vi "csm_lumikki_instron_startLogging_poller.vi"() -> ()   [LabVIEW 2009]
uses:
  <vilib>/Utility/file.llb/Write To Spreadsheet File (DBL).vi
panel:
  in  "Interval/Buffer Parameters":T1={"Sample interval - ms (2)"=2.0, "Buffer Length (1000)"=1000, "No. of Buffers (0)"=0} {"Sample interval - ms (2)" min=0.2 format="%.1f"}
  out "Waveform Graph 2":dbl[][](graph)
  # "datalogger internal \npreferences:"
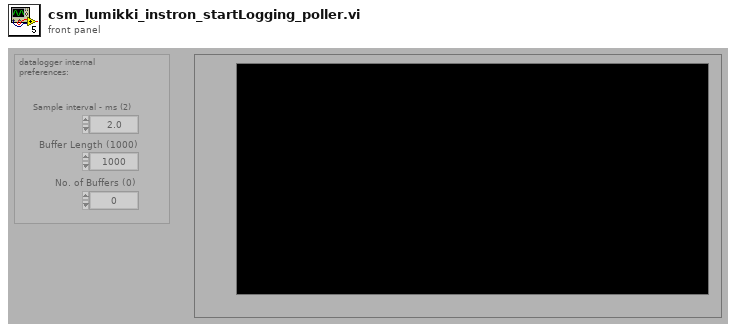
[diagram p1: front panel]
types:
  T1 = cluster{"Sample interval - ms (2)":dbl, "Buffer Length (1000)":i32, "No. of Buffers (0)":i32}
  T2 = cluster{"Device ID":i32, "Device Name":string, "Device Type":i32}[]
  T3 = typedef "NI_Matrix.lvlib/RealMatrix.ctl" = dbl[][]
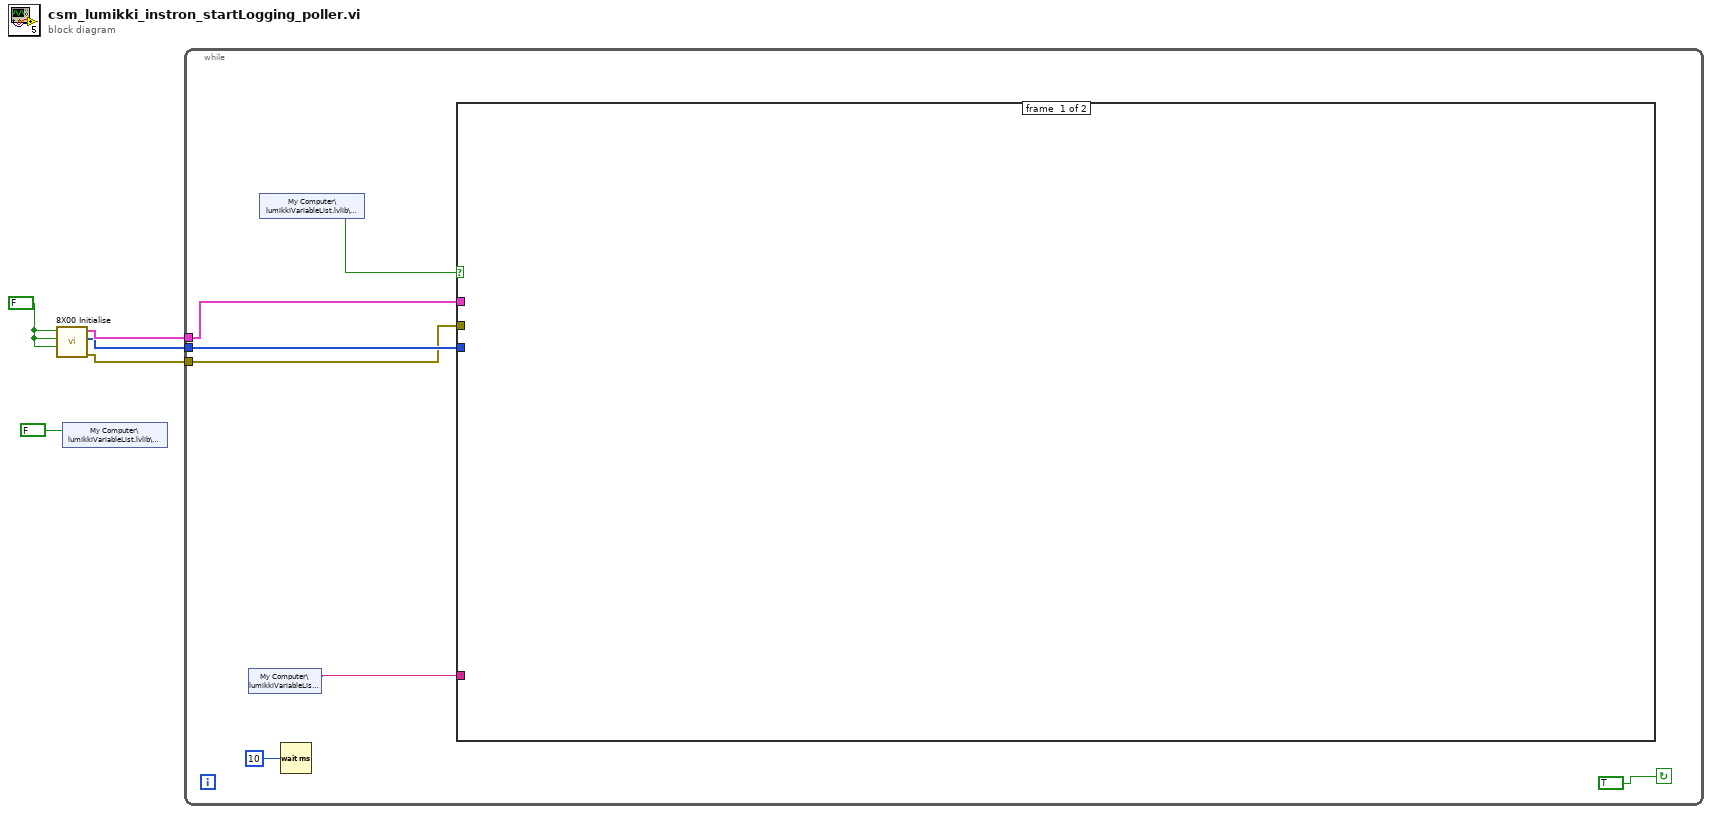
[diagram p0: block diagram]
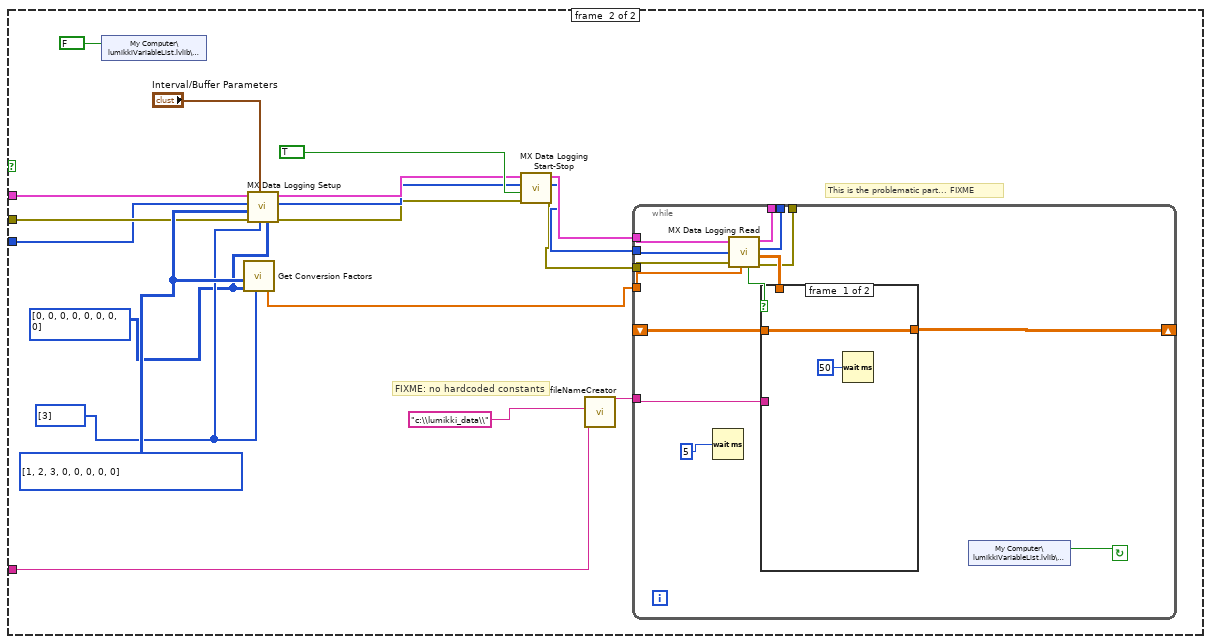
[diagram p2: hidden frame]
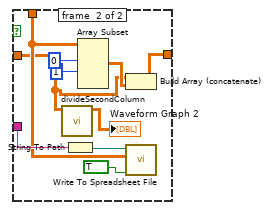
[diagram p3: hidden frame]
diagram:
  w5 = FALSE ("Create Console? (T)")
  n1 = call "8X00 Initialise.vi"("Reset?"=w5, "Create DVM? (T)"=w5, "Create Console? (T)"=w5) -> ("error out"=w2:errorcluster, "Axis Selector"=w3:i32[], "Axis Information"=w4:T2)  [unwired: 1 in, 1 out]
  n2 = shared-variable "My Computer\\lumikkiVariableList.lvlib\\startLogging"(FALSE ("startLogging")) -> ()  [unwired: 1 in, 1 out]
  n3 = while {
    tunnel: w4 -> [w10]
    tunnel: w3 -> [w9]
    tunnel: w2 -> [w8]
    stop <- TRUE continue-if-true
    n4 = shared-variable "My Computer\\lumikkiVariableList.lvlib\\expId"() -> (w6:string)  [unwired: 1 in, 1 out]
    n5 = shared-variable "My Computer\\lumikkiVariableList.lvlib\\startLogging"() -> (w7:bool)  [unwired: 1 in, 1 out]
    n6 = Wait (ms)(milliseconds to wait=u32 10) -> ()  [unwired: 1 out]
    n7 = case shown="True" w7 {
      tunnel: w10 -> [_ w16]
      tunnel: w9 -> [_ w17]
      tunnel: w8 -> [_ w18]
      tunnel: w6 -> [_ w15]
      frame #0 {
      }
      frame #1 {
        w28 = i32[] [3] ("Number of Columns")
        w27 = i32[][] [[0, 0, 0, 0, 0, 0, 0, 0]] items=["Feedback", "Direct Auxilary"] ("Column Types")
        w29 = i32[][] [[1, 2, 3, 0, 0, 0, 0, 0]] items=["Not Used", "Channel 1/Logging time", "Channel 2/Controlling command", "Channel 3/Controlling error", "Channel 4/Elapsed quarter-cycle counter", "Total accumulated quarter-cycle counter", "Elapsed segment counter", "Total accumulated segment counter", "Servovalve drive", "Block count", "Uncompensated servovalve drive", "Geometric compensation output 1", "Geometric compensation output 2", "Re-Sampling Filter 1", "Re-Sampling Filter 2", "Re-Sampling Filter 3", "Re-Sampling Filter 4", "Outer cascaded controller output", "Delta_P or acceleration compensation (Raw)", "Auxiliary input from the front of the IAC", "Waveform identifier", "Reserved", "Digital I/O and sample playback actions", "Reserved", "Motor current (EIB only)", "Motor instantaneous power (EIB only)", "Motot filtered power (EIB only)", "Motor speed (EIB only)", "Motor viscous loss (EIB only)"] ("Column Channels")
        # "FIXME: no hardcoded constants"
        # "This is the problematic part... FIXME"
        n8 = shared-variable "My Computer\\lumikkiVariableList.lvlib\\startLogging"(FALSE ("startLogging")) -> ()  [unwired: 1 in, 1 out]
        n9 = call "Get Conversion Factors.vi"("Column Channels"=w29, "Column Types"=w27, "Number of Columns"=w28) -> ("Conversion Factors"=w30:dbl[])  [unwired: 2 in]
        n10 = call "MX Data Logging Setup.vi"("Column Types"=w27, "Number of Columns"=w28, "Interval/Buffer Parameters"="Interval/Buffer Parameters", "error in (no error)"=w18, "Column Channels"=w29, "Axis Selector"=w17, "Axis Information"=w16) -> ("error out"=w22:errorcluster, "Axis Selector copy"=w23:i32[], "Axis Information out"=w24:T2)  [unwired: 1 out]
        n11 = call "MX Data Logging Start-Stop.vi"("error in (no error)"=w22, "Start (T)"=TRUE, "Axis Selector"=w23, "Axis Information"=w24) -> ("error out"=w19:errorcluster, "Axis Selector copy"=w20:i32[], "Axis Information out"=w21:T2)  [unwired: 4 in]
        n12 = call "fileNameCreator.vi"("folder"="c:\\lumikki_data\\", "Measurement ID"=w15) -> ("concatenated string"=w31:string)  [unwired: 9 in]
        n13 = while {
          tunnel: [w37] -> _
          tunnel: [w38] -> _
          tunnel: w19 -> [w41]
          tunnel: w30 -> [w40]
          tunnel: w20 -> [w42]
          tunnel: w21 -> [w43]
          tunnel: [w36] -> _
          tunnel: w31 -> [w35]
          shift-right: [w34] -> _
          shift-left: _ -> [w33]
          stop <- w32 continue-if-true
          n14 = Wait (ms)(milliseconds to wait=u32 5) -> ()  [unwired: 1 out]
          n15 = call "MX Data Logging Read.vi"("Axis Information"=w43, "Axis Selector"=w42, "error in (no error)"=w41, "Conversion Values (100)"=w40) -> ("Axis Information copy"=w36:T2, "Axis Selector copy"=w38:i32[], "Data Available"=w39:bool, "Collected Data - Eng Units"=w44:dbl[][], "error out"=w37:errorcluster)  [unwired: 2 out]
          n16 = case shown="True" w39 {
            tunnel: w44 -> [_ w54]
            tunnel: w35 -> [_ w55]
            tunnel: [w46 w50] -> w34
            tunnel: w33 -> [w46 w49]
            frame #0 {
              n17 = Wait (ms)(milliseconds to wait=u32 50) -> ()  [unwired: 1 out]
            }
            frame #1 {
              n18 = call "divideSecondColumn.vi"("Real Matrix"=w49) -> ("submatrix"=→"Waveform Graph 2":T3)  [unwired: 10 in]
              n19 = String To Path(string=w55) -> (path=w57:path)
              n20 = Array Subset(array=w54, index (row)=0 ("index"), length (row)=1 ("length")) -> (w51:dbl[][])  [unwired: 2 in]
              n21 = Build Array (concatenate)(w49, w51) -> (w50:dbl[][])
              n22 = call-poly <vilib>:"Write To Spreadsheet File.vi"("append to file? (new file:F)"=TRUE, "2D data"=w54, "file path (dialog if empty)"=w57) -> ()  [unwired: 5 in, 1 out]
            }
          }
          n23 = shared-variable "My Computer\\lumikkiVariableList.lvlib\\loggingIsOn"() -> (w32:bool)  [unwired: 1 in, 1 out]
        }
      }
    }
  }
